vi "Write Flange 2 Width.vi"(8 "error in (no error)":errorcluster, 10 "Flange2Width":u32, 11 "MultiSegmentPipe.lvclass in":refnum<class "MultiSegmentPipe.lvclass">) -> (0 "error out":errorcluster, 3 "MultiSegmentPipe.lvclass out":refnum<class "MultiSegmentPipe.lvclass">)   [LabVIEW 2015, in "MultiSegmentPipe.lvclass"]
uses:
  MultiSegmentPipe.lvclass
  MultiSegmentPipe.lvclass/MultiSegmentPipe.ctl
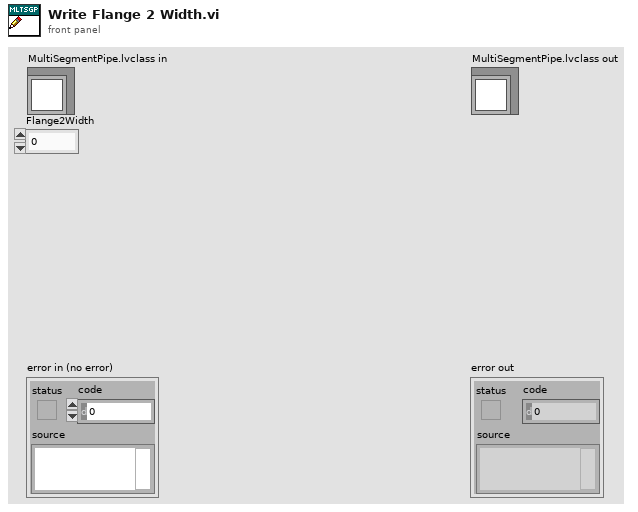
[diagram p1: front panel]
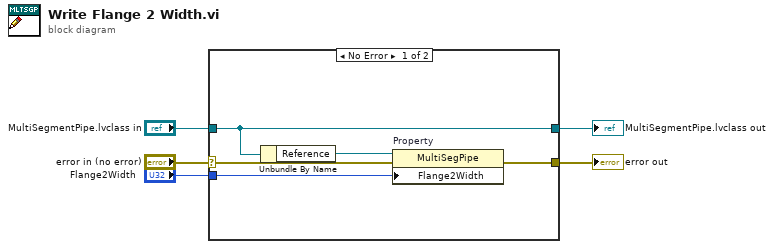
[diagram p0: block diagram]
diagram:
  n1 = case shown="No Error" "error in (no error)" {
    selector: "error in (no error)" -> [w6 w12]
    tunnel: [w10 w12] -> w4
    tunnel: [w8 w11] -> w2
    tunnel: "MultiSegmentPipe.lvclass in" -> [w8 w11]
    tunnel: "Flange2Width" -> [w9 _]
    frame No Error {
      n2 = Unbundle By Name(w8) -> ("Reference"=w7:refnum<vi>)
      n3 = property on="Property" class="MultiSegPipe"(reference=w7, error in=w6, "Flange2Width"=w9) -> (error out=w10:errorcluster)  [unwired: 1 out]
    }
    frame Error {
    }
  }
  "error out" <- w4
  "MultiSegmentPipe.lvclass out" <- w2
